vi "fgv_DWA_config.vi"(7 "cmd":T2, 11 "config":T1={"max speed"=1.0, "min speed"=-0.5, "max yaw rate"=0.0, "max accel"=0.2, "max delta yaw rate"=0.0, "v resolution"=0.01, "yaw rate resolution"=0.1, "dt"=0.1, "predict time"=3.0, "to goal cost gain"=0.15, "speed cost gain"=1.0, "obstacle cost gain"=0.0, "robot stuck flag cons"=0.001, "robot type"=enum."circle", "robot radius"=1.0, "robot width"=0.5, "robot length"=1.2, "obstacles"=[], "goal pt"={"x"=90, "y"=90}}) -> (3 "config out":T1={"max speed"=1.0, "min speed"=-0.5, "max yaw rate"=0.0, "max accel"=0.2, "max delta yaw rate"=0.0, "v resolution"=0.01, "yaw rate resolution"=0.1, "dt"=0.1, "predict time"=3.0, "to goal cost gain"=0.15, "speed cost gain"=1.0, "obstacle cost gain"=0.0, "robot stuck flag cons"=0.001, "robot type"=enum."circle", "robot radius"=1.0, "robot width"=0.5, "robot length"=1.2, "obstacles"=[], "goal pt"={"x"=90, "y"=90}})   [LabVIEW 2019]
uses:
  Ctrl/cmd_common.ctl
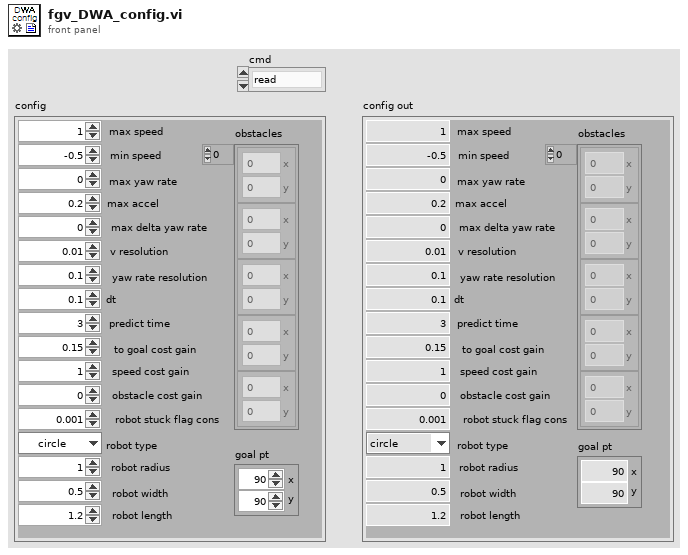
[diagram p1: front panel]
types:
  T1 = cluster{"max speed":dbl, "min speed":dbl, "max yaw rate":dbl, "max accel":dbl, "max delta yaw rate":dbl, "v resolution":dbl, "yaw rate resolution":dbl, "dt":dbl, "predict time":dbl, "to goal cost gain":dbl, "speed cost gain":dbl, "obstacle cost gain":dbl, "robot stuck flag cons":dbl, "robot type":enum16{"circle", "rectangle"}, "robot radius":dbl, "robot width":dbl, "robot length":dbl, "obstacles":cluster{"x":dbl, "y":dbl}[], "goal pt":cluster{"x":i32, "y":i32}}
  T2 = typedef "cmd_common.ctl" = enum16{"read", "write"}
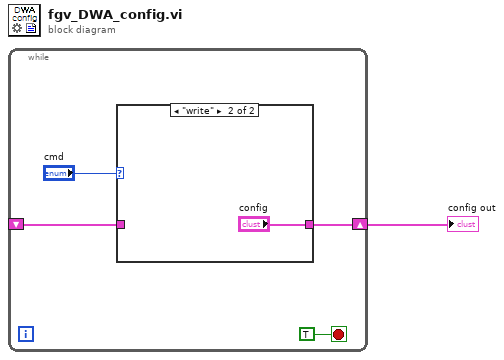
[diagram p0: block diagram]
diagram:
  n1 = while {
    shift-right: [w3] -> w1
    shift-left: _ -> [w2]
    stop <- TRUE stop-if-true
    n2 = case shown="\"write\"" "cmd" {
      tunnel: [w6 "config"] -> w3
      tunnel: w2 -> [w6 _]
      frame "read", Default {
      }
      frame "write" {
      }
    }
  }
  "config out" <- w1
